vi "store states.vi"(6 "counter index":u8, 7 "pulse not yet sent":bool, 9 "next output":bool, 10 "current output":bool) -> (3 "state out":u16)   [LabVIEW 2018, in "trigger-out.lvlib"]
uses:
  trigger-out.lvlib
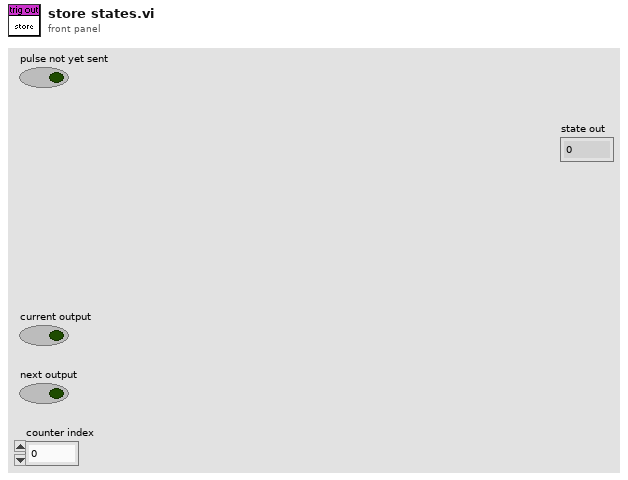
[diagram p1: front panel]
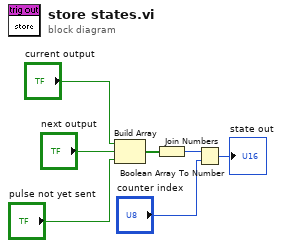
[diagram p0: block diagram]
diagram:
  n1 = Build Array("current output", "next output", "pulse not yet sent") -> (w3:bool[])
  n2 = Boolean Array To Number(Boolean array=w3) -> (number=w2:u8)
  n3 = Join Numbers(hi=w2, lo="counter index") -> ((hi.lo)=→"state out":u16)
